vi "ziModGetAuxinData.vi"(8 "Error In":errorcluster, 10 "ModResults":T3, 11 "ModHandle In":T6 {"ModHandle" format="0x%08x"; "Conn" format="0x%08x"}) -> (0 "Error Out":errorcluster, 1 "AuxInSampleGrid":T1[](array[typedef]), 2 "AuxInSample":T2[](array[typedef]), 3 "ModHandle Out":T6 {"ModHandle" format="0x%08x"; "Conn" format="0x%08x"})   [LabVIEW 2018, in "Zurich Instruments LabOne.lvlib"]
doc: "Use this vi to get AuxIn (node: /DEV*/AUXINS/*/STREAM) Data from a ModResult returned from ziModGetNextNode.vi. It returns an array of AuxIn Data."
uses:
  Zurich Instruments LabOne.lvlib
  ziTypeModHandle.ctl
  ziTypeModResults.ctl
  Data/ziTypePollType.ctl
  ziTypeModGenericHeader.ctl
  Data/ziTypeAuxInSample.ctl
  Data/ziTypeAuxInSampleGrid.ctl
  Data/ziTypeDoubleDataTS.ctl
  ziLV32.dll
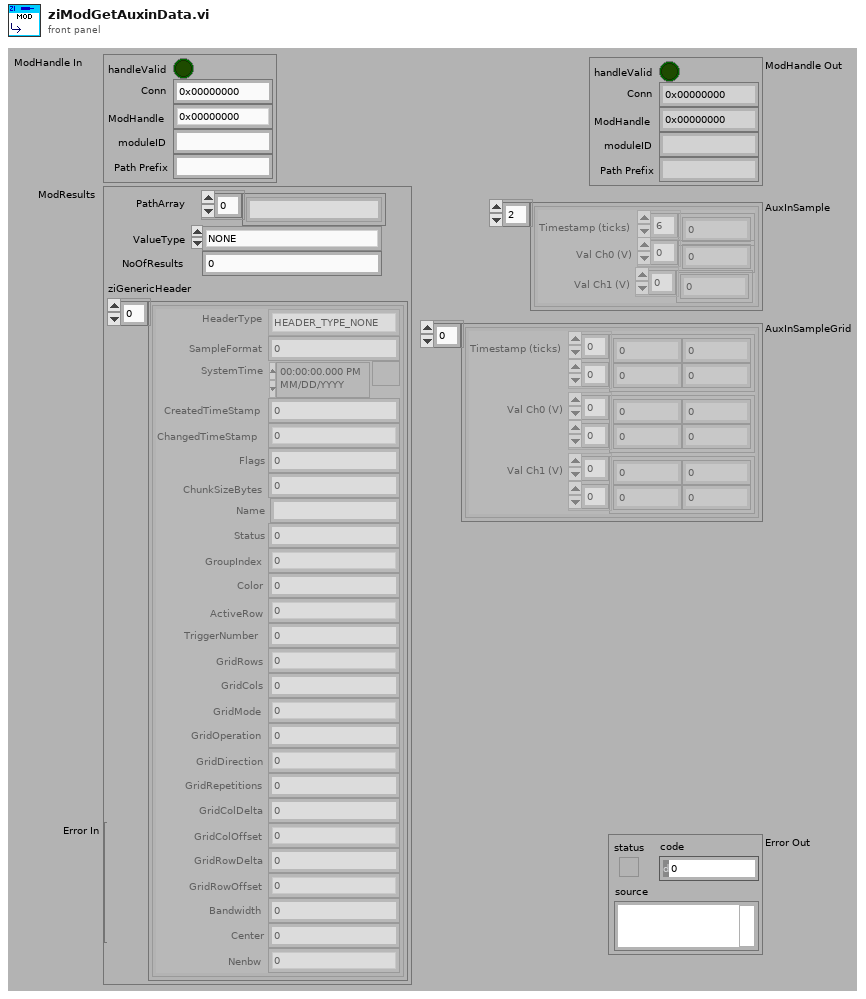
[diagram p1: front panel]
types:
  T1 = typedef "Zurich Instruments LabOne.lvlib/ziTypeAuxInSampleGrid.ctl" = cluster{"Timestamp (ticks)":u64[][], "Val Ch0 (V)":dbl[][], "Val Ch1 (V)":dbl[][]}
  T2 = typedef "Zurich Instruments LabOne.lvlib/ziTypeAuxInSample.ctl" = cluster{"Timestamp (ticks)":u64[], "Val Ch0 (V)":dbl[], "Val Ch1 (V)":dbl[]}
  T3 = typedef "Zurich Instruments LabOne.lvlib/ziTypeModResults.ctl" = cluster{"PathArray":string[], "ValueType":T4, "NoOfResults":u64, "ziGenericHeader":T5[]}
  T4 = typedef "Zurich Instruments LabOne.lvlib/ziTypePollType.ctl" = enum16{"NONE", "DOUBLE_DATA", "INTEGER_DATA", "DEMOD_SAMPLE", "SCOPE_WAVE_HF2", "AUXIN_SAMPLE", "DIO_SAMPLE", "BYTE_ARRAY", "PWA_WAVE", "9", "10", "11", "12", "13", "14", "15", "TREE_CHANGE_DEPRI", "17", "ERROR", "19", "20", "21", "22", "23", "24", "25", "26", "27", "28", "29", "30", "31", "DOUBLE_DATA_TS", "INTEGER_DATA_TS", "34", "SCOPE_WAVE", "SCOPE_WAVE_EX", "37", "BYTE_ARRAY_TS", "39", "40", "41", "42", "43", "44", "45", "CNT_DATA", "47", "TREE_CHANGE", "49", "50", "51", "52", "53", "54", "55", "56", "57", "58", "59", "60", "61", "62", "63", "SWEEPER_DATA", "SPECTRUM_DATA", "ADVISOR_DATA", "VECTOR_DATA", "IMP_DATA"}
  T5 = typedef "Zurich Instruments LabOne.lvlib/ziTypeModGenericHeader.ctl" = cluster{"HeaderType":enum8{"HEADER_TYPE_NONE", "HEADER_TYPE_SWTRIGGER", "HEADER_TYPE_SWEEPER"}, "SampleFormat":u8, "SystemTime":timestamp, "CreatedTimeStamp":u64, "ChangedTimeStamp":u64, "Flags":u32, "ChunkSizeBytes":u64, "Name":string, "Status":u32, "GroupIndex":u32, "Color":u32, "ActiveRow":u32, "TriggerNumber":u64, "GridRows":u32, "GridCols":u32, "GridMode":u32, "GridOperation":u32, "GridDirection":u32, "GridRepetitions":u32, "GridColDelta":dbl, "GridColOffset":dbl, "GridRowDelta":dbl, "GridRowOffset":dbl, "Bandwidth":dbl, "Center":dbl, "Nenbw":dbl}
  T6 = typedef "Zurich Instruments LabOne.lvlib/ziTypeModHandle.ctl" = cluster{"handleValid":bool, "Conn":u64, "ModHandle":u64, "moduleID":string, "Path Prefix":string}
  T7 = typedef "Zurich Instruments LabOne.lvlib/ziTypeDoubleDataTS.ctl" = cluster{"Timestamp (ticks)":u64[], "Value":dbl[]}
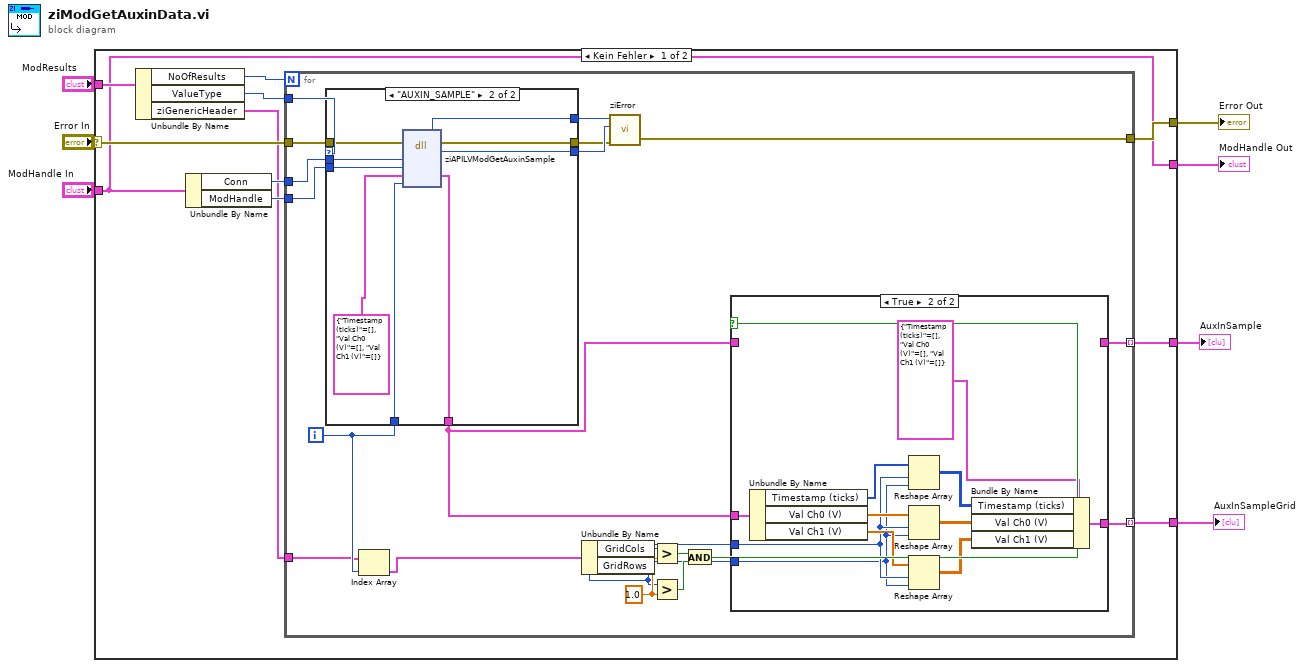
[diagram p0: block diagram]
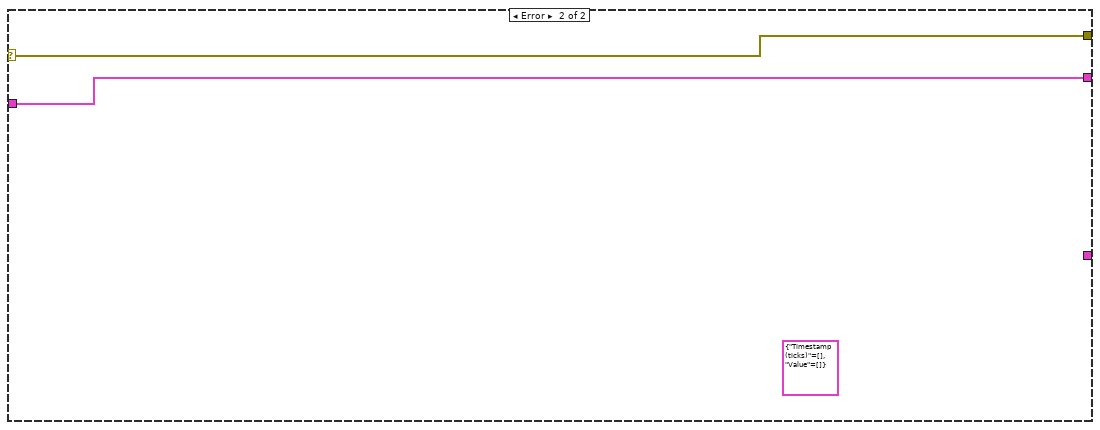
[diagram p4: hidden frame]
diagram:
  n1 = case shown="Kein Fehler" "Error In" {
    selector: "Error In" -> [w13 w62]
    tunnel: [w14 w62] -> w3
    tunnel: [w12 w63] -> w6
    tunnel: "ModHandle In" -> [w12 w63]
    tunnel: "ModResults" -> [w16 _]
    tunnel: [w10 _] -> w2
    tunnel: [w8 _] -> w1
    frame No Error {
      n2 = Unbundle By Name(w16) -> ("NoOfResults"=w15:u64, "ValueType"=w11:T4, "ziGenericHeader"=w9:T5[])
      n3 = Unbundle By Name(w12) -> ("Conn"=w18:u64, "ModHandle"=w17:u64)
      n4 = for {
        N: w15 -> [_]
        tunnel: w18 -> [w38]
        tunnel: w17 -> [w37]
        tunnel: [w36] -> w14
        tunnel: w13 -> [w33]
        tunnel: w11 -> [w32]
        tunnel: [w22] -> w10 mode=indexing
        tunnel: w9 -> [w19]
        tunnel: [w24] -> w8 mode=indexing
        i -> [w20]
        w30 = 1.0 ("y")
        n5 = case shown="\"AUXIN_SAMPLE\"" w32 {
          tunnel: w38 -> [w51 w61]
          tunnel: w37 -> [_ w60]
          tunnel: w20 -> [_ w59]
          tunnel: [_ w58] -> w35
          tunnel: [w52 w57] -> w34
          tunnel: w33 -> [w52 w56]
          tunnel: [_ w55] -> w23
          tunnel: [w51 w53] -> w31
          frame "NONE", Default {
          }
          frame "AUXIN_SAMPLE" {
            n6 = dll-call lib="ziLV*.*" fn="ziAPILVModGetAuxinSample"(error in=w56, "Conn"=w61, "ModHandle"=w60, "AuxInData"=T2 {"Timestamp (ticks)"=[], "Val Ch0 (V)"=[], "Val Ch1 (V)"=[]} ("AuxInput"), "chunk_idx"=w59) -> (error out=w57:errorcluster, "return type"=w58:u32, "Conn"=w53:u64, "AuxInData"=w55:T2)  [unwired: 4 in, 1 out]
          }
        }
        n7 = Index Array(array=w19, index=w20) -> (element=w21:T5)
        n8 = Unbundle By Name(w21) -> ("GridCols"=w25:u32, "GridRows"=w26:u32)
        n9 = call "ziError.vi"("Conn"=w31, "ziErrorCode"=w35, "Error In"=w34) -> ("Error Out"=w36:errorcluster)  [unwired: 2 in, 1 out]
        n10 = Greater?(x=w25, y=w30) -> (0:w28:bool)
        n11 = Greater?(x=w26, y=w30) -> (0:w29:bool)
        n12 = And(x=w28, y=w29) -> (x .and. y?=w27:bool)
        n13 = case shown="True" w27 {
          tunnel: w23 -> [_ w50]
          tunnel: w26 -> [_ w46]
          tunnel: w25 -> [_ w44]
          tunnel: [_ w45] -> w24
          tunnel: w23 -> [w39 _]
          tunnel: [w39 _] -> w22
          frame False {
          }
          frame True {
            n14 = Unbundle By Name(w50) -> ("Timestamp (ticks)"=w49:u64[], "Val Ch0 (V)"=w48:dbl[], "Val Ch1 (V)"=w47:dbl[])
            n15 = Reshape Array(w49, w46, w44) -> (w43:u64[][])
            n16 = Reshape Array(w48, w46, w44) -> (w42:dbl[][])
            n17 = Reshape Array(w47, w46, w44) -> (w41:dbl[][])
            n18 = Bundle By Name(cluster=T1 {"Timestamp (ticks)"=[], "Val Ch0 (V)"=[], "Val Ch1 (V)"=[]} ("AuxInput"), "Timestamp (ticks)"=w43, "Val Ch0 (V)"=w42, "Val Ch1 (V)"=w41) -> (w45:T1)
          }
        }
      }
    }
    frame Error {
      (unwired) T7 {"Timestamp (ticks)"=[], "Value"=[]} ("DoubleSample")
    }
  }
  "Error Out" <- w3
  "ModHandle Out" <- w6
  "AuxInSample" <- w2
  "AuxInSampleGrid" <- w1
